vi "LowLvCtrl_Loop.vi"(8 "error in (no error)":errorcluster, 9 "LoadCell Task":refnum<k21>="LoadCells_AI", 10 "FPGA VI Reference In":refnum<k20>, 11 "MotorCtrl In":refnum<class "MotorControl.lvclass">) -> (0 "error out":errorcluster, 1 "LoadCell Task dup":refnum<k21>="LoadCells_AI", 2 "FPGA VI Reference Out":refnum<k20>, 3 "MotorCtrl Out":refnum<class "MotorControl.lvclass">)   [LabVIEW 2015]
uses:
  Classes/MotorControl/MotorControl.lvclass
  <vilib>/Platform/TimedLoop/XDataNode/timing_clust.ctl
  <vilib>/Platform/TimedLoop/XDataNode/nitl_modes.ctl
  <vilib>/Platform/TimedLoop/XDataNode/wakeup.ctl
  Classes/MotorControl/TypeDef/MotorMode.ctl
  <vilib>/DAQmx/read.llb/DAQmx Read (Analog 1D Wfm NChan NSamp).vi
  <vilib>/Analysis/baseanly.llb/Mean (DBL).vi
  <vilib>/DAQmx/miscellaneous.llb/DAQmx Fill In Error Info.vi
  <vilib>/measure/macond.llb/IIR Filter for N Chan.vi
  <vilib>/Utility/error.llb/Error Cluster From Error Code.vi
  <vilib>/rvi/errors/niLvFpgaAdjustHostInterfaceError.vi
  <vilib>/Platform/TimedLoop/XDataNode/XDataNode.xnode
  <vilib>/rvi/interface/nirviReadWriteControl/nirviReadWriteControl.xnode
  <vilib>/Platform/TimedLoop/XDataNode/XDNodeRunTimeDep.lvlib
  <vilib>/measure/NI_MAPro.lvlib
  <vilib>/Analysis/NI_AALBase.lvlib
  <vilib>/rvi/interface/Simulation/niFpgaSimulationCallBeginRW.vi
  NiFpgaLv.dll
  Shared Libraries/CustomVIs/CustomVI.lvlib
panel:
  in  "Friction Compensation(F)":bool
  in  "Analog Input Filter":T1={"Topology"=enum."Butterworth", "Type"=enum."Lowpass", "Order"=1, "Lower Fc"=30.0, "Upper Fc"=200.0, "PB Ripple"=1.0, "SB Attenuation"=60.0} {"PB Ripple" format="%0.2f"; "SB Attenuation" format="%0.2f"; "Lower Fc" format="%0.2p"; "Upper Fc" format="%0.2p"}
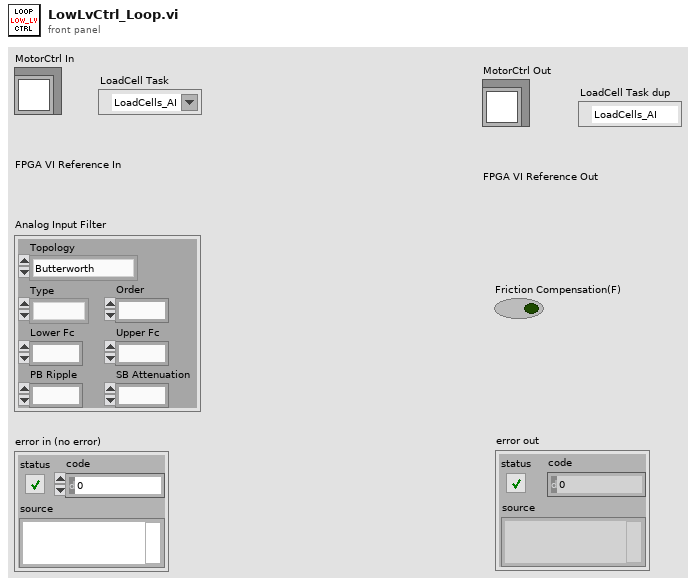
[diagram p1: front panel]
types:
  T1 = cluster{"Topology":enum16{"Off", "Butterworth", "Chebyshev", "Inverse Chebyshev", "Elliptic", "Bessel"}, "Type":enum16{"Lowpass", "Highpass", "Bandpass", "Bandstop"}, "Order":i32, "Lower Fc":dbl, "Upper Fc":dbl, "PB Ripple":dbl, "SB Attenuation":dbl}
  T2 = typedef "XDNodeRunTimeDep.lvlib/timing_clust.ctl" = cluster{"Expected End [f-1]":u64, "Actual End [f-1]":u64, "Finished Late? [f-1]":bool, "Expected End [i-1]":u64, "Actual End [i-1]":u64, "Finished Late? [i-1]":bool, "Expected Start [i]":u64, "Actual Start [i]":u64, "Expected Start [f]":u64, "Actual Start [f]":u64, "Source Name":string, "Structure Name":string, "Period":i64, "Deadline":i64, "Offset":i64, "Start":i64, "Priority":i32, "Timeout":i32, "Mode":T3, "Wakeup Reason":T4, "Error":errorcluster, "Source Type":string, "Secondary Source Type":string, "Global End Time":u64, "Global Start Time":u64, "Frame Duration":u64, "Iteration Duration":u64, "Assigned CPU":i32, "I/O Scan Engine Mode":u32}
  T3 = typedef "XDNodeRunTimeDep.lvlib/nitl_modes.ctl" = enum32{"No Change", "Process missed periods, maintain original phase", "Discard missed periods, maintain original phase", "Process missed periods, ignore original phase", "Discard missed periods, ignore original phase"}
  T4 = typedef "XDNodeRunTimeDep.lvlib/wakeup.ctl" = enum32{"Normal", "Aborted", "Asynchronous wakeup", "Timing source error", "Timed loop error", "Timeout"}
  T5 = cluster{"Input":enum16{"Fr:Cable", "Fr:Motor", "Fr:Sensor"}, "Output":enum16{"To:Cable", "To:Motor", "To:Sensor"}}
  T6 = typedef "MotorControl.lvclass/MotorMode.ctl" = enum16{"Idle", "FF", "PID"}
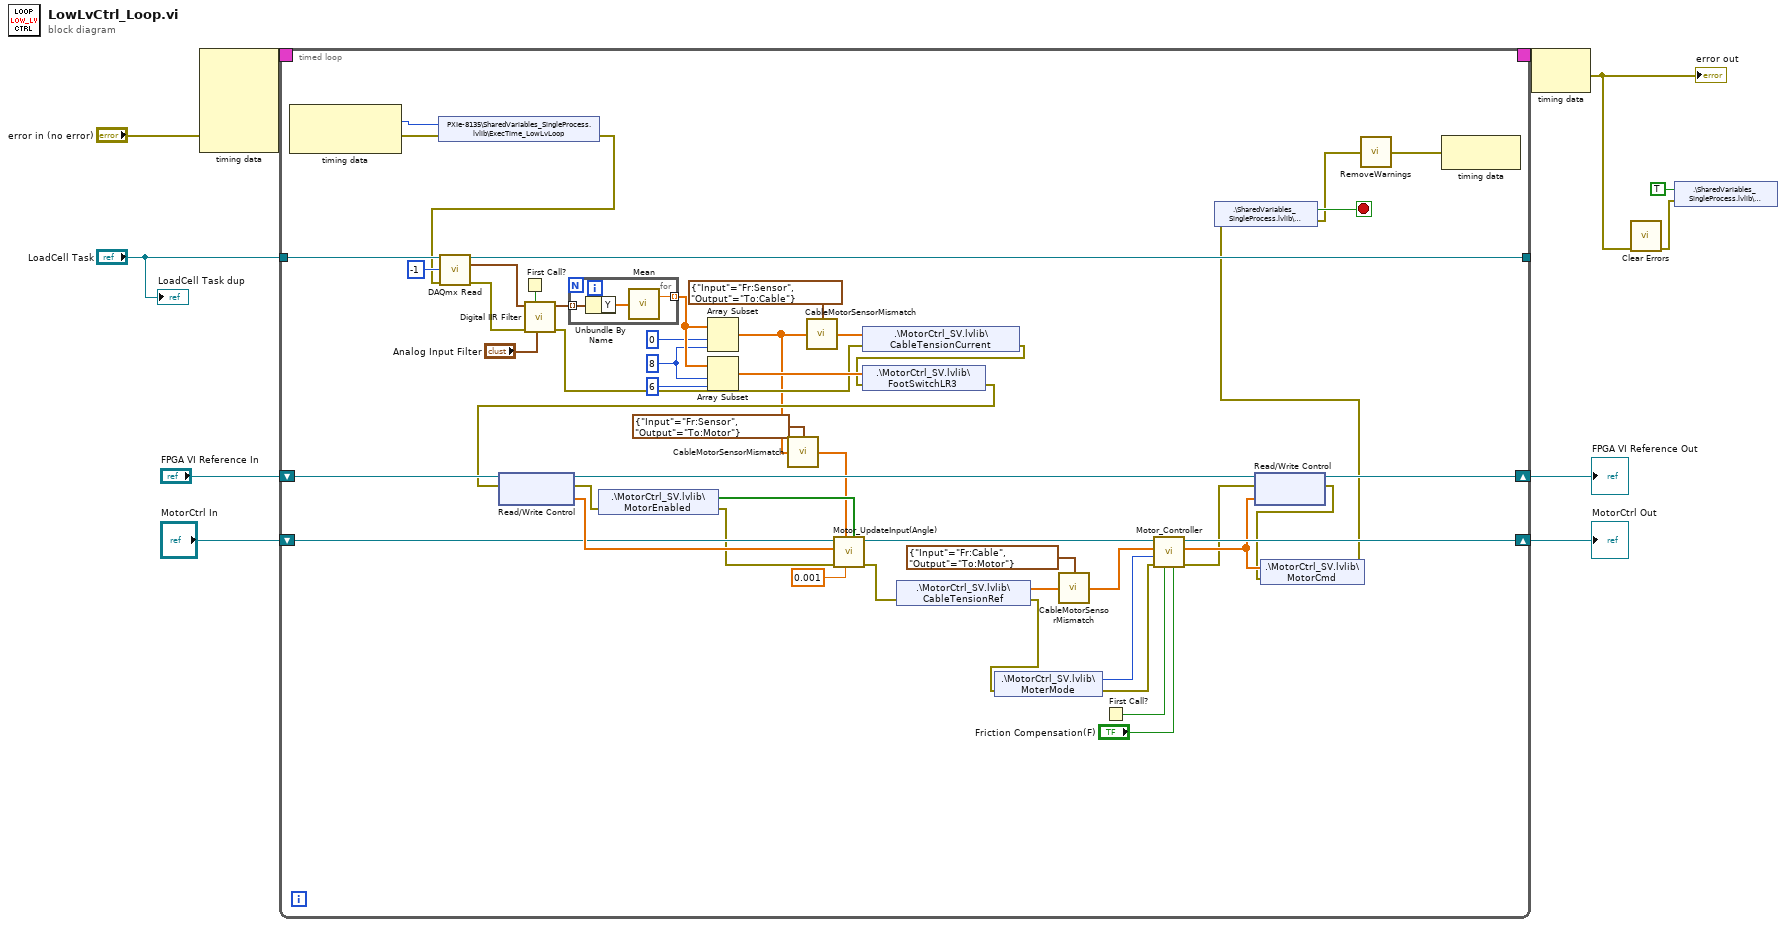
[diagram p0: block diagram]
diagram:
  n1 = node-c288("error in (no error)") -> (w11:T2)  [unwired: 4 in]
  n2 = timed-loop {
    timing: w11 -> [_]
    timing-out: [_] -> w10
    tunnel: "LoadCell Task" -> [w62]
    tunnel: [w51] -> _
    shift-right: [w47] -> w8
    shift-left: "MotorCtrl In" -> [w52]
    shift-right: [w45] -> w5
    shift-left: "FPGA VI Reference In" -> [w54]
    stop <- w33 stop-if-true
    w41 = 8 ("length")
    n3 = node-c288() -> (w37:i64, w32:errorcluster)  [unwired: 1 in]
    n4 = shared-variable "PXIe-8135\\SharedVariables_SingleProcess.lvlib\\ExecTime_LowLvLoop"(w37, error in=w32) -> (error out=w31:errorcluster)
    n5 = call-poly <vilib>:"DAQmx Read.vi"("task/channels in"=w62, "number of samples per channel"=-1, "error in"=w31) -> ("task out"=w51:refnum<k21>, "data"=w60:waveform(dbl)[], "error out"=w59:errorcluster)  [unwired: 10 in]
    n6 = First Call?() -> (First Call?: T/F=w58:bool)
    n7 = call-poly <vilib>:"Digital IIR Filter.vi"("IIR filter specifications"="Analog Input Filter", "reset filters"=w58, "error in (no error)"=w59, "signal(s) in"=w60) -> ("error out"=w28:errorcluster, "signal(s) out"=w56:waveform(dbl)[])  [unwired: 5 in, 1 out]
    n8 = for {
      tunnel: w56 -> [w65] mode=indexing
      tunnel: [w63] -> w42 mode=indexing
      n9 = Unbundle By Name(w65) -> ("Y"=w64:dbl[])
      n10 = call-poly <vilib>:"Mean.vi"("X"=w64) -> ("mean"=w63:dbl)  [unwired: 1 out]
    }
    n11 = Array Subset(array=w42, index=0 ("length"), length=w41) -> (w21:dbl[])
    n12 = Array Subset(array=w42, index=w41, length=6) -> (w40:dbl[])
    n13 = call "CableMotorSensorMismatch.vi"("Conversion"=T5 {"Input"=enum."Fr:Sensor", "Output"=enum."To:Motor"}, "Input"=w21) -> ("Output"=w22:dbl[])  [unwired: 2 in]
    n14 = call "CableMotorSensorMismatch.vi"("Conversion"=T5 {"Input"=enum."Fr:Sensor", "Output"=enum."To:Cable"}, "Input"=w21) -> ("Output"=w20:dbl[])  [unwired: 2 in]
    n15 = shared-variable ".\\MotorCtrl_SV.lvlib\\CableTensionCurrent"(w20, error in=w28) -> (error out=w30:errorcluster)
    n16 = shared-variable ".\\MotorCtrl_SV.lvlib\\FootSwitchLR3"(w40, error in=w30) -> (error out=w29:errorcluster)
    n17 = xnode "Read/Write Control"("FPGA VI Reference In"=w54, "error in"=w29) -> ("FPGA VI Reference Out"=w46:refnum<k20>, "error out"=w35:errorcluster, "EncdAngle"=w53:sgl[])
    n18 = shared-variable ".\\MotorCtrl_SV.lvlib\\MotorEnabled"(error in=w35) -> (w43:bool[], error out=w34:errorcluster)
    n19 = call "Motor_UpdateInput(Angle).vi"("Enabled"=w43, "dt (for angle derivitive)"=0.001, "CableTensionNow(N)"=w22, "error in (no error)"=w34, "MotorEncAngle(rad)"=w53, "Motor in"=w52) -> ("error out"=w27:errorcluster, "Motor out"=w55:refnum<class "MotorControl.lvclass">)  [unwired: 4 in]
    n20 = shared-variable ".\\MotorCtrl_SV.lvlib\\CableTensionRef"(error in=w27) -> (w19:dbl[], error out=w26:errorcluster)
    n21 = shared-variable ".\\MotorCtrl_SV.lvlib\\MoterMode"(error in=w26) -> (w48:T6, error out=w25:errorcluster)
    n22 = call "CableMotorSensorMismatch.vi"("Conversion"=T5 {"Input"=enum."Fr:Cable", "Output"=enum."To:Motor"}, "Input"=w19) -> ("Output"=w18:dbl[])  [unwired: 2 in]
    n23 = First Call?() -> (First Call?: T/F=w49:bool)
    n24 = call "Motor_Controller.vi"("Friction Compensation(F)"="Friction Compensation(F)", "Reinitialize? (F)"=w49, "error in (no error)"=w25, "Mode"=w48, "CableTensionRef(N)"=w18, "Motor in"=w55) -> ("error out"=w36:errorcluster, "VoltageCommand"=w44:dbl[], "Motor out"=w47:refnum<class "MotorControl.lvclass">)  [unwired: 3 in]
    n25 = xnode "Read/Write Control"("FPGA VI Reference In"=w46, "error in"=w36, "AmpCmd"=w44) -> ("FPGA VI Reference Out"=w45:refnum<k20>, "error out"=w24:errorcluster)
    n26 = shared-variable ".\\MotorCtrl_SV.lvlib\\MotorCmd"(w44, error in=w24) -> (error out=w23:errorcluster)
    n27 = shared-variable ".\\SharedVariables_SingleProcess.lvlib\\GlobalStop"(error in=w23) -> (w33:bool, error out=w12:errorcluster)
    n28 = call "RemoveWarnings.vi"("error in (no error)"=w12) -> ("error out"=w13:errorcluster)
    n29 = node-c288(w13) -> ()  [unwired: 1 out]
  }
  "MotorCtrl Out" <- w8
  "FPGA VI Reference Out" <- w5
  n30 = node-c288(w10) -> (w2:errorcluster)
  "error out" <- w2
  n31 = call <vilib>:"Clear Errors.vi"("error in (no error)"=w2) -> ("error out"=w1:errorcluster)  [unwired: 5 in, 1 out]
  n32 = shared-variable ".\\SharedVariables_SingleProcess.lvlib\\GlobalStop"(TRUE ("GlobalStop"), error in=w1) -> ()  [unwired: 1 out]
  "LoadCell Task dup" <- "LoadCell Task"
